vi "calcStiffnesses.vi"(8 "error in (no error)":errorcluster, 11 "Model in":refnum<class "Model.lvclass">) -> (0 "error out":errorcluster, 3 "Model out":refnum<class "Model.lvclass">)   [LabVIEW 2015, in "Model.lvclass"]
uses:
  Model.lvclass
  Typedefs/StiffnessDataAssembly.ctl
  Typedefs/StiffnessData.ctl
  Typedefs/StiffnessesDataSummary.ctl
  Model.lvclass/Model.ctl
  UserEvents/UserEvents.lvclass/UserEvents.ctl
  ApplicationElements/StiffnessCalculator/StiffnessCalculator.lvclass/StiffnessCalculator.ctl
  ApplicationElements/Log/TestDataLog/TestDataLog.lvclass/TestDataLog.ctl
  ApplicationElements/StiffnessCalculator/StiffnessCalculator.lvclass
  ApplicationElements/Log/TestDataLog/TestDataLog.lvclass
  UserEvents/UserEvents.lvclass
  Typedefs/M1M3SSSTypedefs.lvlib
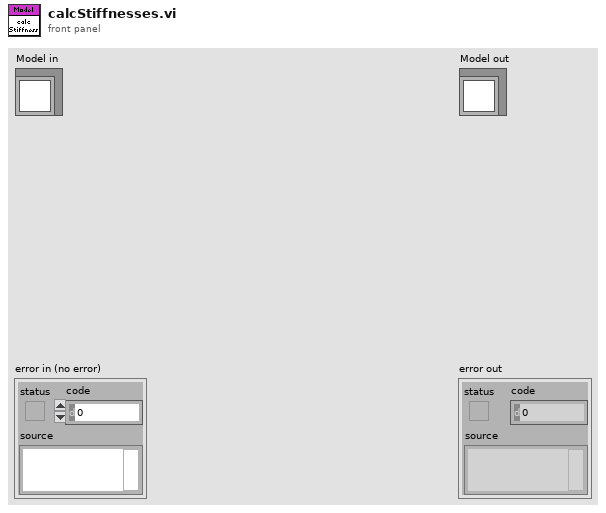
[diagram p1: front panel]
types:
  T1 = typedef "M1M3SSSTypedefs.lvlib/StiffnessDataAssembly.ctl" = cluster{"Stiffness Data":T2, "Stiffnesses Data Summary":T3, "graph file path":path}
  T2 = typedef "M1M3SSSTypedefs.lvlib/StiffnessData.ctl" = cluster{"Distance Measured":dbl[unit][], "Force Measured":dbl[unit][]}
  T3 = typedef "M1M3SSSTypedefs.lvlib/StiffnessesDataSummary.ctl" = cluster{"Forces":dbl[unit][], "Displacements":dbl[unit][], "Stiffnesses":dbl[unit][]}
  T4 = typedef "M1M3SSSTypedefs.lvlib/PubDataEvents.ctl" = cluster{"State":refnum<user-event>, "ErrorCode":refnum<user-event>, "OutputData":refnum<user-event>, "InputData":refnum<user-event>, "ControllerData":refnum<user-event>, "TestStatus":refnum<user-event>, "LogPath":refnum<user-event>, "StiffnessDataAssembly":refnum<user-event>, "PreconditioningCycle":refnum<user-event>}
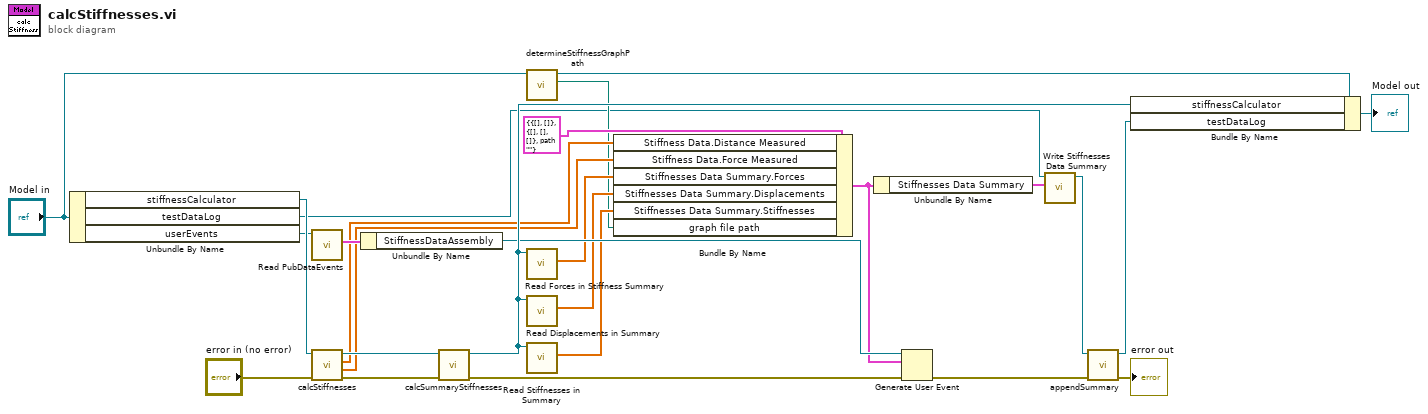
[diagram p0: block diagram]
diagram:
  n1 = Unbundle By Name("Model in") -> ("stiffnessCalculator"=w26:refnum<class "StiffnessCalculator.lvclass">, "testDataLog"=w1:refnum<class "TestDataLog.lvclass">, "userEvents"=w21:refnum<class "UserEvents.lvclass">)
  n2 = call "Read PubDataEvents.vi"("UserEvents in"=w21) -> ("PubDataEvents"=w16:T4)  [unwired: 9 in, 1 out]
  n3 = call "calcStiffnesses.vi"("error in (no error)"="error in (no error)", "StiffnessCalculator in"=w26) -> ("error out"=w13:errorcluster, "forceMeasuredArray"=w10:dbl[unit][], "distanceMeasuredArray"=w11:dbl[unit][], "StiffnessCalculator out"=w25:refnum<class "StiffnessCalculator.lvclass">)  [unwired: 6 in]
  n4 = Unbundle By Name(w16) -> ("StiffnessDataAssembly"=w17:refnum<user-event>)
  n5 = call "calcSummaryStiffnesses.vi"("error in (no error)"=w13, "StiffnessCalculator in"=w25) -> ("error out"=w15:errorcluster, "StiffnessCalculator out"=w22:refnum<class "StiffnessCalculator.lvclass">)  [unwired: 8 in]
  n6 = call "determineStiffnessGraphPath.vi"("Model in"="Model in") -> ("graph file path"=w2:path, "Model out"=w3:refnum<class "Model.lvclass">)  [unwired: 8 in, 1 out]
  n7 = call "Read Forces in Stiffness Summary.vi"("StiffnessCalculator in"=w22) -> ("Forces in Stiffness Summary"=w9:dbl[unit][])  [unwired: 9 in, 1 out]
  n8 = call "Read Displacements in Summary.vi"("StiffnessCalculator in"=w22) -> ("Displacements in Summary"=w8:dbl[unit][])  [unwired: 9 in, 1 out]
  n9 = call "Read Stiffnesses in Summary.vi"("StiffnessCalculator in"=w22) -> ("Stiffnesses in Summary"=w7:dbl[unit][])  [unwired: 9 in, 1 out]
  n10 = Bundle By Name(cluster=T1 {"Stiffness Data"={"Distance Measured"=[], "Force Measured"=[]}, "Stiffnesses Data Summary"={"Forces"=[], "Displacements"=[], "Stiffnesses"=[]}, "graph file path"=path ""} ("StiffnessDataAssembly"), "Stiffness Data.Distance Measured"=w11, "Stiffness Data.Force Measured"=w10, "Stiffnesses Data Summary.Forces"=w9, "Stiffnesses Data Summary.Displacements"=w8, "Stiffnesses Data Summary.Stiffnesses"=w7, "graph file path"=w2) -> (w6:T1)
  n11 = Unbundle By Name(w6) -> ("Stiffnesses Data Summary"=w5:T3)
  n12 = Generate User Event(user event=w17, event data cluster=w6, error in=w15) -> (error out=w14:errorcluster)  [unwired: 1 in, 1 out]
  n13 = call "Write Stiffnesses Data Summary.vi"("Stiffnesses Data Summary"=w5, "TestDataLog in"=w1) -> ("TestDataLog out"=w20:refnum<class "TestDataLog.lvclass">)  [unwired: 9 in]
  n14 = call "appendSummary.vi"("error in (no error)"=w14, "TestDataLog in"=w20) -> ("error out"=→"error out":errorcluster, "TestDataLog out"=w19:refnum<class "TestDataLog.lvclass">)  [unwired: 8 in]
  n15 = Bundle By Name(cluster=w3, "stiffnessCalculator"=w22, "testDataLog"=w19) -> (→"Model out":refnum<class "Model.lvclass">)
